vi "plan_stp_motion.vi"(2 "error in (no error)":errorcluster caption="错误输入（无错误）", 3 "init? (T)":bool=TRUE, 4 "stp":dbl, 5 "OneMotion 输入":refnum<class "OneMotion.lvclass">) -> (0 "error out":errorcluster caption="错误输出", 1 "OneMotion 输出":refnum<class "OneMotion.lvclass">)   [LabVIEW 2016, in "MotionControl_UFO_3DOF.lvlib" / "OneMotion.lvclass"]
uses:
  <userlib>/MotionControl_UFO_3DOF/OneMotion/OneMotion.lvclass
  <userlib>/MotionControl_UFO_3DOF/OneMotion/OneMotion.lvclass/OneMotion.ctl
  <userlib>/MotionControl_UFO_3DOF/OneMotion/cmd_motion.ctl
  <userlib>/MotionControl_UFO_3DOF/MotionControl_UFO_3DOF.lvlib
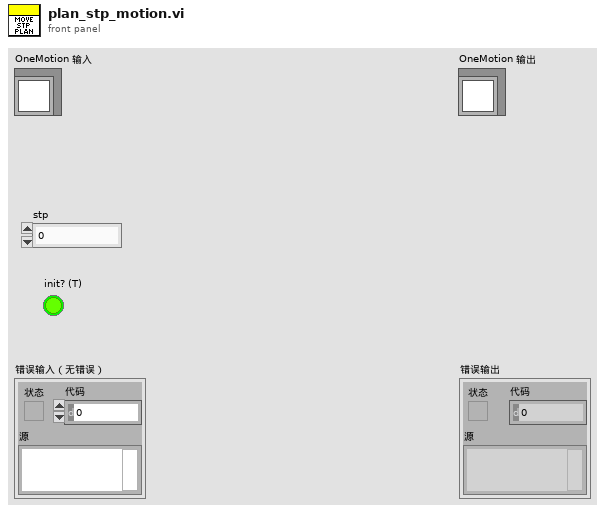
[diagram p1: front panel]
types:
  T1 = typedef "MotionControl_UFO_3DOF.lvlib/OneMotion.lvclass/cmd_motion.ctl" = enum16{"NONE", "MOVE_MOTION", "EXIT", "STP_MOTION", "SPEED_MOTION", "WAIT_FOR_S3", "WAIT_A_TIME", "SKIP", "RETRACT_BEFORE_ROT"}
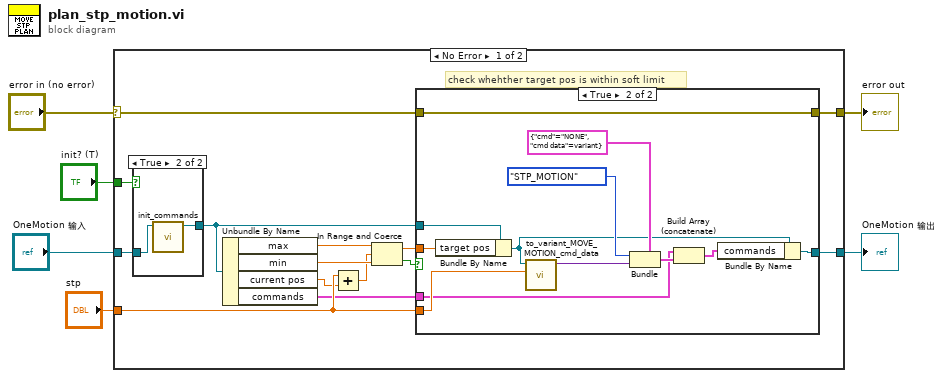
[diagram p0: block diagram]
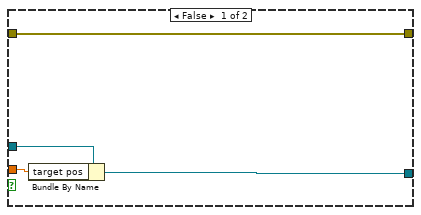
[diagram p3: hidden frame]
diagram:
  n1 = case shown="No Error" "error in (no error)" {
    selector: "error in (no error)" -> [w19 w41]
    tunnel: [w18 w41] -> w5
    tunnel: [w20 w40] -> w4
    tunnel: "OneMotion 输入" -> [w8 w40]
    tunnel: "stp" -> [w17 _]
    tunnel: "init? (T)" -> [w9 _]
    frame No Error {
      # "check whehther target pos is within soft limit"
      n2 = case shown="True" w9 {
        tunnel: w8 -> [w21 w23]
        tunnel: [w21 w22] -> w7
        frame False {
        }
        frame True {
          n3 = call-dynamic "init_commands.vi"("OneMotion 输入"=w23) -> ("OneMotion 输出"=w22:refnum<class "OneMotion.lvclass">)  [unwired: 9 in, 1 out]
        }
      }
      n4 = Unbundle By Name(w7) -> ("max"=w16:dbl, "min"=w13:dbl, "current pos"=w12:dbl, "commands"=w10:cluster{"cmd":T1, "cmd data":variant}[])
      n5 = Add(x=w17, y=w12) -> (x+y=w11:dbl)
      n6 = In Range and Coerce(upper limit=w16, x=w11, lower limit=w13) -> (coerced(x)=w14:dbl, In Range?=w15:bool)
      n7 = case shown="True" w15 {
        tunnel: w7 -> [w27 w39]
        tunnel: w14 -> [w26 w29]
        tunnel: [w25 w37] -> w20
        tunnel: w17 -> [_ w38]
        tunnel: w19 -> [w24 w36]
        tunnel: [w24 w36] -> w18
        tunnel: w10 -> [_ w28]
        frame False {
          n8 = Bundle By Name(cluster=w27, "target pos"=w26) -> (w25:refnum<class "OneMotion.lvclass">)
        }
        frame True {
          n9 = Bundle By Name(cluster=w39, "target pos"=w29) -> (w32:refnum<class "OneMotion.lvclass">)
          n10 = call <userlib>:"to_variant_MOVE_MOTION_cmd_data.vi"("target pos"=w38, "OneMotion.lvclass"=w32) -> ("variant"=w31:variant)  [unwired: 9 in]
          n11 = Bundle(cluster=cluster{"cmd":T1, "cmd data":variant} {"cmd"=enum."NONE", "cmd data"=variant} ("command cluster"), "cmd"=cmd_motion."STP_MOTION", "cmd data"=w31) -> (w30:cluster{"cmd":T1, "cmd data":variant})
          n12 = Build Array (concatenate)(w28, w30) -> (w35:cluster{"cmd":T1, "cmd data":variant}[])
          n13 = Bundle By Name(cluster=w32, "commands"=w35) -> (w37:refnum<class "OneMotion.lvclass">)
        }
      }
    }
    frame Error {
    }
  }
  "error out" <- w5
  "OneMotion 输出" <- w4
